vi "Append VI List of SubVIs to Report (path).vi"(0 "report in":refnum<class "NI_report.lvclass">, 2 "image format (jpeg)":enum32{"PNG", "JPEG", "GIF"}(ring)=enum."JPEG", 5 "VI":path, 7 "alignment (default)":T2, 9 "include Express VI configuration information (F)":bool, 11 "error in (no error)":errorcluster, 12 "MS Office parameters":T1) -> (4 "report out":refnum<class "NI_report.lvclass">, 6 "VI path out":path, 8 "start out (Word)":i32, 10 "end out (Word)":i32, 15 "error out":errorcluster)   [LabVIEW 2017, in "NI_ReportGenerationCore.lvlib"]
doc: "Appends a list of subVIs of the VI you specify in <B>VI</B> to a report. The list includes subVI icons, names, and paths. Wire data to the <B>VI</B> input to determine the polymorphic instance to use or manually select the instance."
uses:
  <vilib>/Utility/NIReport.llb/NI_ReportGenerationCore.lvlib
  <vilib>/Utility/NIReport.llb/NI_report.lvclass
  <vilib>/Utility/NIReport.llb/HTML Report Image Alignment.ctl
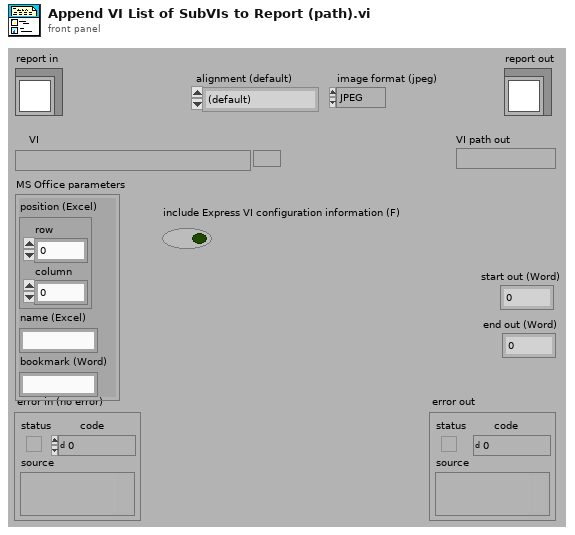
[diagram p1: front panel]
types:
  T1 = cluster{"position (Excel)":cluster{"row":i32, "column":i32}, "name (Excel)":string, "bookmark (Word)":string}
  T2 = typedef "NI_ReportGenerationCore.lvlib/HTML Report Image Alignment.ctl" = enum16{"(default)", "LEFT", "RIGHT", "TOP", "TEXTTOP", "MIDDLE", "ABSMIDDLE", "BASELINE", "BOTTOM", "ABSBOTTOM"}
  T3 = enum32{"invalid app kind", "Development System", "Run Time System", "Student Edition", "Embedded LabVIEW", "Evaluation", "Custom"}
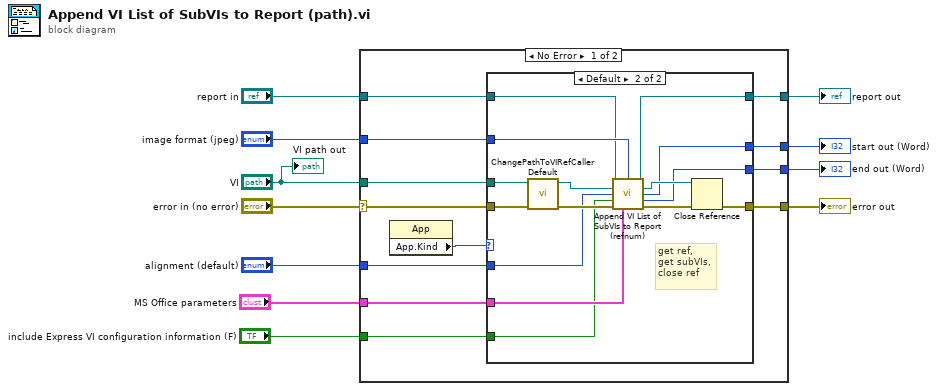
[diagram p0: block diagram]
diagram:
  n1 = case shown="No Error" "error in (no error)" {
    selector: "error in (no error)" -> [w23 w42]
    tunnel: [w19 w42] -> w10
    tunnel: [w13 w41] -> w8
    tunnel: "report in" -> [w14 w41]
    tunnel: "VI" -> [w16 _]
    tunnel: "image format (jpeg)" -> [w20 _]
    tunnel: "alignment (default)" -> [w22 _]
    tunnel: "MS Office parameters" -> [w21 _]
    tunnel: [w18 _] -> w3
    tunnel: [w17 _] -> w2
    tunnel: "include Express VI configuration information (F)" -> [w15 _]
    frame No Error {
      n2 = property class="App"() -> ("App.Kind"=w12:T3)  [unwired: 2 in, 2 out]
      n3 = case shown="Default" w12 {
        tunnel: w23 -> [w25 w40]
        tunnel: w22 -> [_ w38]
        tunnel: w21 -> [_ w37]
        tunnel: w20 -> [_ w36]
        tunnel: [w25 w34] -> w19
        tunnel: [_ w27] -> w18
        tunnel: [_ w26] -> w17
        tunnel: w16 -> [_ w32]
        tunnel: w15 -> [_ w30]
        tunnel: w14 -> [w24 w29]
        tunnel: [w24 w28] -> w13
        frame "Run Time System" {
          # "Do not try to append\nif running in an\nexecutable"
        }
        frame Default {
          # "get ref,\nget subVIs,\nclose ref"
          n4 = call <vilib>:"ChangePathToVIRefCallerDefault.vi"("error in (no error)"=w40, "VI path"=w32) -> ("error out"=w39:errorcluster, "VI reference"=w31:refnum<vi>)  [unwired: 4 out]
          n5 = call <vilib>:"Append VI List of SubVIs to Report (refnum).vi"("report in"=w29, "image format (jpeg)"=w36, "VI"=w31, "alignment (default)"=w38, "include Express VI configuration information (F)"=w30, "error in (no error)"=w39, "MS Office parameters"=w37) -> ("report out"=w28:refnum<class "NI_report.lvclass">, "VI out"=w33:refnum<vi>, "start out (Word)"=w27:i32, "end out (Word)"=w26:i32, "error out"=w35:errorcluster)  [unwired: 1 in, 3 out]
          n6 = Close Reference(reference=w33, error in (no error)=w35) -> (error out=w34:errorcluster)
        }
      }
    }
    frame Error {
    }
  }
  "error out" <- w10
  "report out" <- w8
  "start out (Word)" <- w3
  "end out (Word)" <- w2
  "VI path out" <- "VI"
